vi "JoinFloatChannel.vi"(11 "Array":dbl[](array[numeric])) -> (3 "OutArray":u8[](array[numeric]))   [LabVIEW 2019]
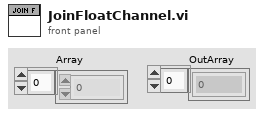
[diagram p1: front panel]
types:
  T1 = enum16{"big-endian, network order", "native, host order", "little-endian"}
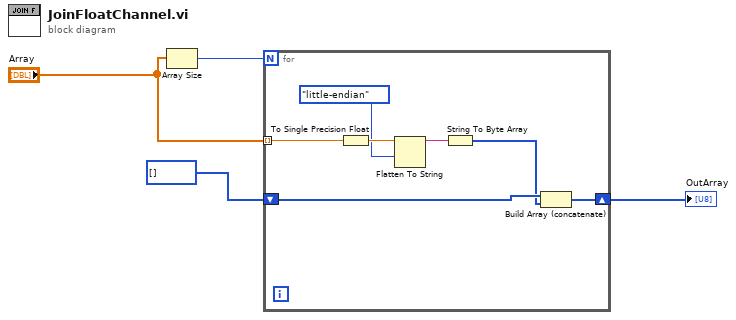
[diagram p0: block diagram]
diagram:
  n1 = Array Size(array="Array") -> (size(s)=w4:i32)
  n2 = for {
    N: w4 -> [_]
    shift-right: [w11] -> w1
    shift-left: u8[] [] -> [w10]
    tunnel: "Array" -> [w9] mode=indexing
    n3 = To Single Precision Float(number=w9) -> (single precision float=w8:sgl)
    n4 = Flatten To String(anything=w8, byte order (0:big-endian, network order)=T1."little-endian") -> (data string=w7:string)  [unwired: 2 in, 2 out]
    n5 = String To Byte Array(string=w7) -> (unsigned byte array=w6:u8[])
    n6 = Build Array (concatenate)(w10, w6) -> (w11:u8[])
  }
  "OutArray" <- w1
